vi "Teleop.vi"(10 "Match Info":T1={"Autonomous Elapsed Seconds"=0.0, "TeleOp Elapsed Seconds"=0.0, "Disabled Elapsed Seconds"=0.0, "Visited Autonomous"=FALSE, "Visited TeleOp"=FALSE, "Visited Disabled"=FALSE, "Autonomous Settings"={"Autonomous Style"=enum."Independent", "VI Refnum"=refnum}}, 11 "Call Context":T2) -> ()   [LabVIEW 2020]
doc: "This VI is called for each TeleOp packet received from the DS where the robot is not disabled. It is often used to read from the joysticks and update I/O or to update setpoints for timed control loops. It should complete and return within 20 milliseconds or it may miss DS packets."
uses:
  <vilib>/Rock Robotics/WPI/DriverStation/WPI_DriverStationDerivedRobotMode.ctl
  <vilib>/Rock Robotics/WPI/DriverStation/WPI_DriverStationMatch Info.ctl
  <vilib>/Rock Robotics/WPI/Solenoid/WPI_SolenoidValue.ctl
  <vilib>/Rock Robotics/Network Tables/NT Read Boolean.vi
  <vilib>/Rock Robotics/Network Tables/NT Read Number.vi
  <vilib>/Rock Robotics/WPI/Utilities/WPI_GetSetVariantRefNum.vi
  <vilib>/Rock Robotics/Network Tables/NT Write Numeric Array.vi
  <vilib>/Rock Robotics/Network Tables/NT Write Boolean Array.vi
  <vilib>/Rock Robotics/WPI/RobotDrive/WPI_RobotDriveArcadeDrive_Standard(NoSaturation).vi
  <vilib>/Rock Robotics/Network Tables/NT Write Boolean.vi
  <vilib>/Rock Robotics/WPI/Solenoid/WPI_SolenoidSetEnum.vi
panel:
  out "Sample Slider 0":dbl(slide) scale=0.0..5.0
  out "Sample Boolean 1":bool
  out "Sample Boolean 0":bool
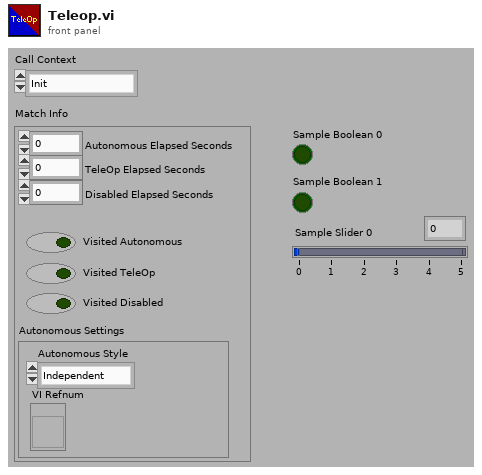
[diagram p1: front panel]
types:
  T1 = typedef "WPI_DriverStationMatch Info.ctl" = cluster{"Autonomous Elapsed Seconds":dbl, "TeleOp Elapsed Seconds":dbl, "Disabled Elapsed Seconds":dbl, "Visited Autonomous":bool, "Visited TeleOp":bool, "Visited Disabled":bool, "Autonomous Settings":cluster{"Autonomous Style":enum16{"Iterative", "Independent"}, "VI Refnum":refnum<vi>}}
  T2 = typedef "WPI_DriverStationDerivedRobotMode.ctl" = enum16{"Init", "Execute", "Stop"}
  T3 = typedef "WPI_SolenoidValue.ctl" = enum16{"Off", "On", "Forward", "Reverse"}
  T4 = typedef "WPI_JoystickDevRef.ctl" = cluster{"Device":T5}
  T5 = typedef "WPI_JoystickDeviceEnum.ctl" = enum16{"USB 0", "USB 1", "USB 2", "USB 3", "USB 4", "USB 5"}
  T6 = cluster{"Axes[0]":dbl, "Axes[1]":dbl, "Axes[2]":dbl, "Axes[3]":dbl, "Axes[4]":dbl, "Axes[5]":dbl, "Axes[6]":dbl, "Axes[7]":dbl, "Axes[8]":dbl}
  T7 = cluster{"Buttons[0]":bool, "Buttons[1]":bool, "Buttons[2]":bool, "Buttons[3]":bool, "Buttons[4]":bool, "Buttons[5]":bool, "Buttons[6]":bool, "Buttons[7]":bool, "Buttons[8]":bool}
  T8 = typedef "WPI_MotorControlDeviceRef.ctl" = cluster{"DeviceStatus":errorcluster, "Type":T9, "PWM":cluster{"PWM Channel":T10, "DeadBand":T11}, "CAN":cluster{"Device Number":u8, "SetOutput VI Ref":variant, "GetOutput VI Ref":variant, "Enable VI Ref":variant, "Disable VI Ref":variant, "Data":variant}, "Invert":bool, "DIO PWM":cluster{"PWM \"Enable\" Channel":T10, "DIOChannel":T12, "PWM Rate":dbl}}
  T9 = typedef "WPI_MotorControlType.ctl" = enum16{"PWM", "CAN", "DIO PWM"}
  T10 = typedef "FPGA_DIOPWMChannel.ctl" = enum8{"PWM 0", "PWM 1", "PWM 2", "PWM 3", "PWM 4", "PWM 5", "PWM 6", "PWM 7", "PWM 8", "PWM 9", "PWM MXP 0", "PWM MXP 1", "PWM MXP 2", "PWM MXP 3", "PWM MXP 4", "PWM MXP 5", "PWM MXP 6", "PWM MXP 7", "PWM MXP 8", "PWM MXP 9", "Invalid"}
  T11 = typedef "WPI_PWMDeadband.ctl" = cluster{"Name":string, "maxPositivePwm":i32, "minPositivePwm":i32, "centerPwm":i32, "maxNegativePwm":i32, "minNegativePwm":i32, "angularRange":u16}
  T12 = typedef "FPGA_DIOChannel.ctl" = enum8{"DIO 0", "DIO 1", "DIO 2", "DIO 3", "DIO 4", "DIO 5", "DIO 6", "DIO 7", "DIO 8", "DIO 9", "DIO MXP 0", "DIO MXP 1", "DIO MXP 2", "DIO MXP 3", "DIO MXP 4", "DIO MXP 5", "DIO MXP 6", "DIO MXP 7", "DIO MXP 8", "DIO MXP 9", "DIO MXP 10", "DIO MXP 11", "DIO MXP 12", "DIO MXP 13", "DIO MXP 14", "DIO MXP 15", "SPI Port CS1", "SPI Port CS2", "SPI Port CS3", "SPI Port MISO", "SPI Port MOSI", "Invalid"}
  T13 = typedef "WPI_SolenoidDevRef.ctl" = cluster{"DevStatus":errorcluster, "Pneumatics Control Module":u8, "Forward Solenoid Channel":T14, "Reverse Solenoid Channel":T14}
  T14 = typedef "WPI_SolenoidChannel.ctl" = enum8{"Solenoid 0", "Solenoid 1", "Solenoid 2", "Solenoid 3", "Solenoid 4", "Solenoid 5", "Solenoid 6", "Solenoid 7", "Solenoid 8", "Solenoid 9", "Solenoid 10", "Solenoid 11", "Solenoid 12", "Solenoid 13", "Solenoid 14", "Solenoid 15", "Invalid"}
  T15 = typedef "WPI_RobotDriveDevRef.ctl" = cluster{"DevStatus":errorcluster, "Motors[]":T8[], "Square Inputs":bool, "Max Output":dbl}
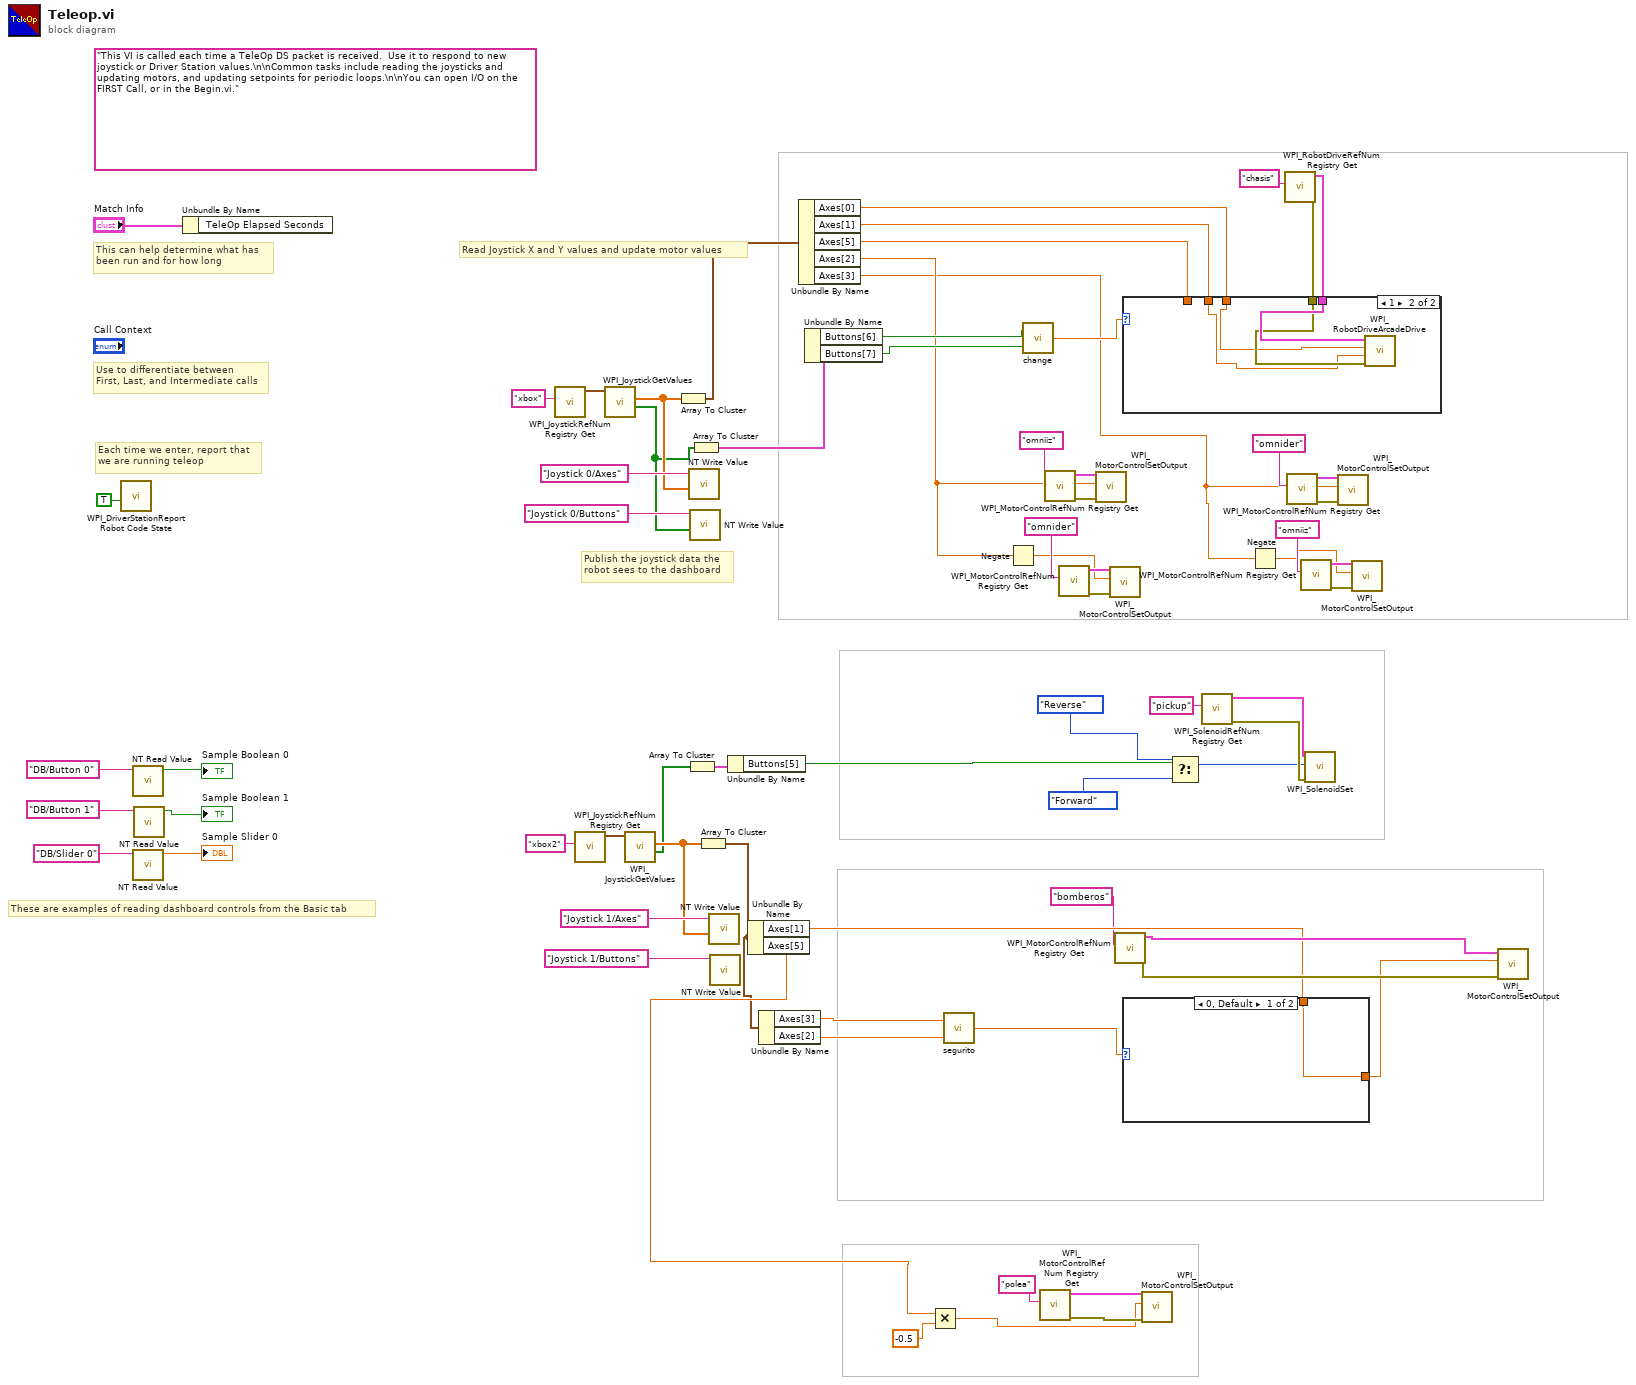
[diagram p0: block diagram]
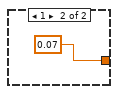
[diagram p2: hidden frame]
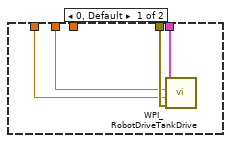
[diagram p3: hidden frame]
diagram:
  (unwired) "This VI is called each time a TeleOp DS packet is received.  Use it to respond to new joystick or Driver Station values.\n\nCommon tasks include reading the joysticks and updating motors, and updating setpoints for periodic loops.\n\nYou can open I/O on the FIRST Call, or in the Begin.vi."
  # "These are examples of reading dashboard controls from the Basic tab"
  # "Publish the joystick data the\nrobot sees to the dashboard"
  # "Each time we enter, report that\nwe are running teleop"
  # "Use to differentiate between\nFirst, Last, and Intermediate calls"
  # "This can help determine what has\nbeen run and for how long"
  # "Read Joystick X and Y values and update motor values"
  n1 = call <vilib>:"WPI_DriverStationReport Robot Code State.vi"("TeleOp"=TRUE ("Autonomous")) -> ()  [unwired: 10 in, 1 out]
  n2 = call-poly <vilib>:"NT Read Value.vi"("Name"="DB/Button 0" ("refnum name")) -> ("Boolean"=→"Sample Boolean 0":bool)  [unwired: 9 in, 1 out]
  n3 = call-poly <vilib>:"NT Read Value.vi"("Name"="DB/Slider 0" ("refnum name")) -> ("Numeric"=→"Sample Slider 0":dbl)  [unwired: 9 in, 1 out]
  n4 = call-poly <vilib>:"NT Read Value.vi"("Name"="DB/Button 1" ("refnum name")) -> ("Boolean"=→"Sample Boolean 1":bool)  [unwired: 9 in, 1 out]
  n5 = Unbundle By Name("Match Info") -> ()  [unwired: 1 out]
  n6 = call <vilib>:"WPI_JoystickRefNum Registry Get.vi"("refnum name"="xbox") -> ("JoystickDevRef"=w69:T4)  [unwired: 1 in, 9 out]
  n7 = call <vilib>:"WPI_JoystickRefNum Registry Get.vi"("refnum name"="xbox2") -> ("JoystickDevRef"=w36:T4)  [unwired: 1 in, 9 out]
  n8 = call <vilib>:"WPI_JoystickGetValues.vi"("JoystickDevRef"=w69) -> ("Buttons"=w46:bool[], "Axes"=w50:dbl[])  [unwired: 6 in, 3 out]
  n9 = call <vilib>:"WPI_JoystickGetValues.vi"("JoystickDevRef"=w36) -> ("Buttons"=w26:bool[], "Axes"=w33:dbl[])  [unwired: 6 in, 3 out]
  n10 = Array To Cluster(array=w50) -> (cluster=w49:T6)
  n11 = Array To Cluster(array=w26) -> (cluster=w31:T7)
  n12 = call-poly <vilib>:"NT Write Value.vi"("Numeric Array"=w50, "Name"="Joystick 0/Axes") -> ()  [unwired: 9 in, 1 out]
  n13 = call-poly <vilib>:"NT Write Value.vi"("Boolean Array"=w46, "Name"="Joystick 0/Buttons") -> ()  [unwired: 9 in, 1 out]
  n14 = Array To Cluster(array=w46) -> (cluster=w45:T7)
  n15 = Array To Cluster(array=w33) -> (cluster=w20:T6)
  n16 = call-poly <vilib>:"NT Write Value.vi"("Numeric Array"=w33, "Name"="Joystick 1/Axes") -> ()  [unwired: 9 in, 1 out]
  n17 = call-poly <vilib>:"NT Write Value.vi"("Name"="Joystick 1/Buttons") -> ()  [unwired: 10 in, 1 out]
  n18 = Unbundle By Name(w31) -> ("Buttons[5]"=w30:bool)
  n19 = Unbundle By Name(w20) -> ("Axes[1]"=w27:dbl, "Axes[5]"=w22:dbl)
  n20 = Unbundle By Name(w20) -> ("Axes[3]"=w19:dbl, "Axes[2]"=w18:dbl)
  n21 = Unbundle By Name(w49) -> ("Axes[0]"=w37:dbl, "Axes[1]"=w39:dbl, "Axes[5]"=w40:dbl, "Axes[2]"=w13:dbl, "Axes[3]"=w1:dbl)
  n22 = Unbundle By Name(w45) -> ("Buttons[6]"=w44:bool, "Buttons[7]"=w43:bool)
  n23 = Multiply(x=w22, y=-0.5) -> (x*y=w21:dbl)
  n24 = call "segurito.vi"("start"=w18, "change"=w19) -> ("output"=w17:dbl)
  n25 = Negate(x=w13) -> (-x=w9:dbl)
  n26 = call "change.vi"("start"=w43, "back"=w44) -> ("output"=w42:dbl)
  n27 = call <vilib>:"WPI_MotorControlRefNum Registry Get.vi"("refnum name"="polea") -> ("error out"=w51:errorcluster, "MotorControlDevRef"=w52:T8)  [unwired: 9 in]
  n28 = call <vilib>:"WPI_MotorControlRefNum Registry Get.vi"("refnum name"="omniiz") -> ("error out"=w16:errorcluster, "MotorControlDevRef"=w15:T8)  [unwired: 9 in]
  n29 = call <vilib>:"WPI_MotorControlRefNum Registry Get.vi"("refnum name"="omnider") -> ("error out"=w12:errorcluster, "MotorControlDevRef"=w11:T8)  [unwired: 9 in]
  n30 = call <vilib>:"WPI_MotorControlSetOutput.vi"("error in (no error)"=w16, "Output"=w13, "MotorControlDevRef"=w15) -> ()  [unwired: 6 in, 3 out]
  n31 = call <vilib>:"WPI_MotorControlSetOutput.vi"("error in (no error)"=w12, "Output"=w9, "MotorControlDevRef"=w11) -> ()  [unwired: 6 in, 3 out]
  n32 = call <vilib>:"WPI_MotorControlRefNum Registry Get.vi"("refnum name"="bomberos") -> ("error out"=w28:errorcluster, "MotorControlDevRef"=w29:T8)  [unwired: 9 in]
  n33 = case shown="0, Default" w17 {
    tunnel: [w71 0.07] -> w25
    tunnel: w27 -> [w71 _]
    frame 0, Default {
    }
    frame 1 {
    }
  }
  n34 = call <vilib>:"WPI_MotorControlSetOutput.vi"("error in (no error)"=w51, "Output"=w21, "MotorControlDevRef"=w52) -> ()  [unwired: 6 in, 3 out]
  n35 = Select(t=WPI_SolenoidValue."Reverse" ("Value"), s=w30, f=WPI_SolenoidValue."Forward" ("Value")) -> (s? t:f=w55:T3)
  n36 = call <vilib>:"WPI_SolenoidRefNum Registry Get.vi"("refnum name"="pickup") -> ("error out"=w58:errorcluster, "SolenoidDevRef"=w59:T13)  [unwired: 9 in]
  n37 = Negate(x=w1) -> (-x=w2:dbl)
  n38 = call <vilib>:"WPI_RobotDriveRefNum Registry Get.vi"("refnum name"="chasis") -> ("error out"=w41:errorcluster, "RobotDriveDevRef"=w38:T15)  [unwired: 9 in]
  n39 = case shown="1" w42 {
    tunnel: w41 -> [w76 w79]
    tunnel: w40 -> [w73 _]
    tunnel: w39 -> [w74 w77]
    tunnel: w38 -> [w75 w80]
    tunnel: w37 -> [_ w78]
    frame 0, Default {
      n40 = call <vilib>:"WPI_RobotDriveTankDrive.vi"("error in (no error)"=w76, "Right axis value"=w73, "Left axis value"=w74, "RobotDriveDevRef"=w75) -> ()  [unwired: 5 in, 3 out]
    }
    frame 1 {
      n41 = call-poly <vilib>:"WPI_RobotDriveArcadeDrive.vi"("error in (no error)"=w79, "Y axis value"=w77, "X axis value"=w78, "RobotDriveDevRef"=w80) -> ()  [unwired: 5 in, 3 out]
    }
  }
  n42 = call <vilib>:"WPI_MotorControlRefNum Registry Get.vi"("refnum name"="omnider") -> ("error out"=w8:errorcluster, "MotorControlDevRef"=w7:T8)  [unwired: 9 in]
  n43 = call <vilib>:"WPI_MotorControlRefNum Registry Get.vi"("refnum name"="omniiz") -> ("error out"=w5:errorcluster, "MotorControlDevRef"=w4:T8)  [unwired: 9 in]
  n44 = call-poly <vilib>:"WPI_SolenoidSet.vi"("error in (no error)"=w58, "Value"=w55, "SolenoidDevRef"=w59) -> ()  [unwired: 7 in, 2 out]
  n45 = call <vilib>:"WPI_MotorControlSetOutput.vi"("error in (no error)"=w8, "Output"=w1, "MotorControlDevRef"=w7) -> ()  [unwired: 6 in, 3 out]
  n46 = call <vilib>:"WPI_MotorControlSetOutput.vi"("error in (no error)"=w5, "Output"=w2, "MotorControlDevRef"=w4) -> ()  [unwired: 6 in, 3 out]
  n47 = call <vilib>:"WPI_MotorControlSetOutput.vi"("error in (no error)"=w28, "Output"=w25, "MotorControlDevRef"=w29) -> ()  [unwired: 6 in, 3 out]
